vi "Watch.vi"(8 "error in (no error)":errorcluster, 11 "QuWire in":refnum<class "QuWire.lvclass">) -> (0 "error out":errorcluster, 3 "QuWire out":refnum<class "QuWire.lvclass">)   [LabVIEW 2020, in "QuWire.lvclass"]
uses:
  QuWire.lvclass
  QuWire.lvclass/QuWire.ctl
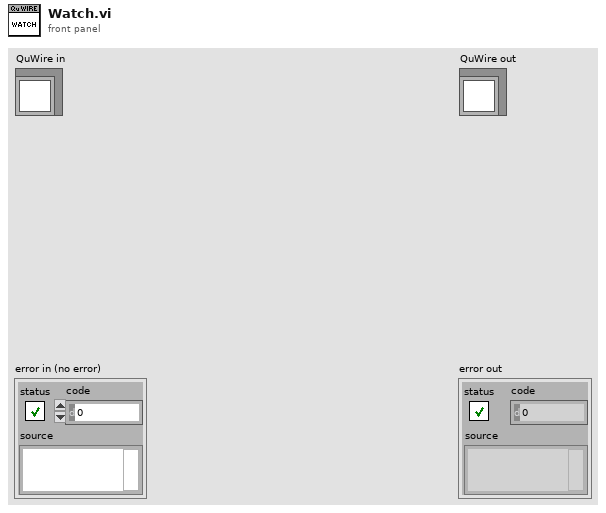
[diagram p1: front panel]
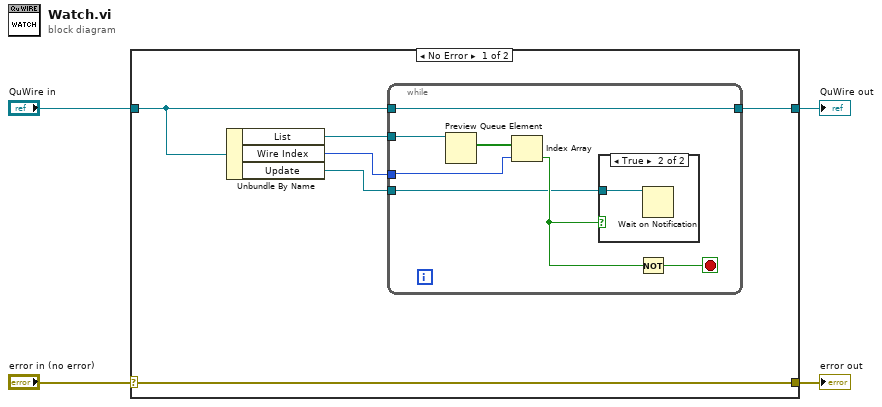
[diagram p0: block diagram]
diagram:
  n1 = case shown="No Error" "error in (no error)" {
    selector: "error in (no error)" -> [w10 w20]
    tunnel: [w10 w20] -> w3
    tunnel: [w5 w19] -> w1
    tunnel: "QuWire in" -> [w6 w19]
    frame No Error {
      n2 = Unbundle By Name(w6) -> ("List"=w8:refnum<queue>, "Wire Index"=w7:i32, "Update"=w9:refnum<notifier>)
      n3 = while {
        tunnel: w7 -> [w16]
        tunnel: w8 -> [w14]
        tunnel: w9 -> [w12]
        tunnel: [w11] -> w5
        tunnel: w6 -> [w11]
        stop <- w15 stop-if-true
        n4 = Preview Queue Element(queue=w14) -> (element=w17:bool[])  [unwired: 2 in, 3 out]
        n5 = Index Array(array=w17, index=w16) -> (element=w13:bool)
        n6 = case shown="True" w13 {
          tunnel: w12 -> [_ w18]
          frame False {
          }
          frame True {
            n7 = Wait on Notification(notifier=w18) -> ()  [unwired: 3 in, 4 out]
          }
        }
        n8 = Not(x=w13) -> (.not. x?=w15:bool)
      }
    }
    frame Error {
    }
  }
  "error out" <- w3
  "QuWire out" <- w1
